vi "GDSLvClass_ReadClassColors.vi"(0 "Library Refnum":refnum<vi>, 5 "error in (no error)":errorcluster) -> (14 "Library Refnum":refnum<vi>, 15 "LvClassIconSettings":T1={"Frame"=0, "Frame thickness"=3, "Header Background"=8453954, "Header Text"=0, "ColorPublic"=16121600, "ColorProtected"=16777215, "ColorPrivate"=16777215, "Body Text"=0, "ClassBodyIcon"=""} {"Frame thickness" min=1 max=3 step=1}, 16 "LvClassIconSettingsFound":bool, 17 "ClassItemIconName(NoExtension)":string, 18 "Type":enum16{"LvClass", "Library", "X-Control"}(ring), 19 "error out":errorcluster)   [LabVIEW 2016]
uses:
  <resource>/Framework/Providers/Open_GDS/ClassProviders/Common/LvClass_class/GDSLvClass_IconSettingsType.ctl
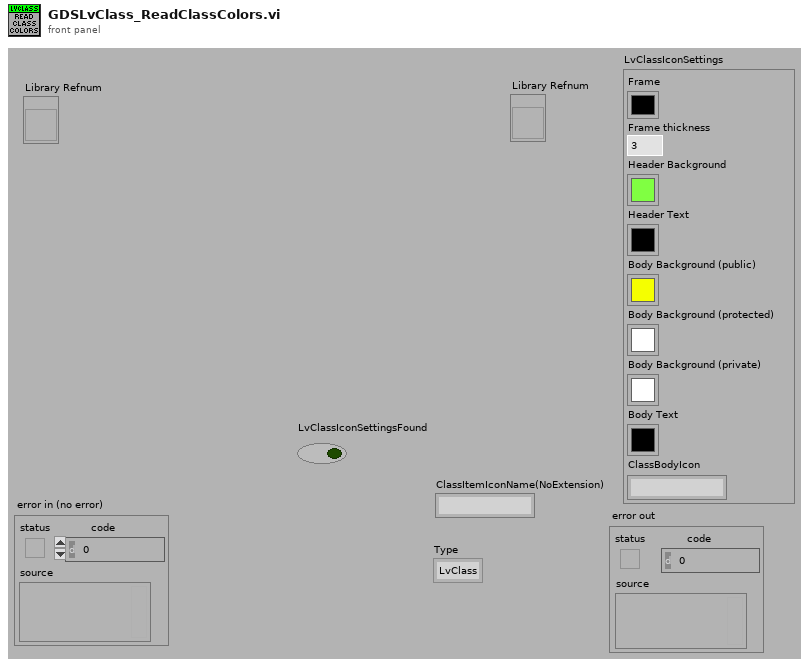
[diagram p1: front panel]
types:
  T1 = typedef "GDSLvClass_IconSettingsType.ctl" = cluster{"Frame":u32, "Frame thickness":u8, "Header Background":u32, "Header Text":u32, "ColorPublic":u32, "ColorProtected":u32, "ColorPrivate":u32, "Body Text":u32, "ClassBodyIcon":string}
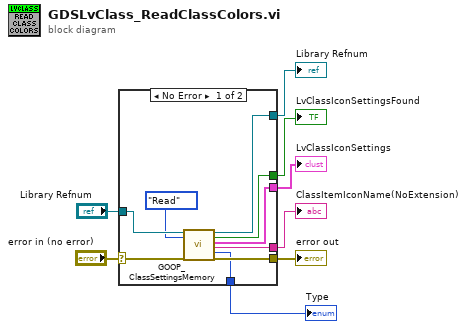
[diagram p0: block diagram]
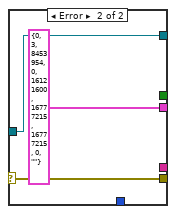
[diagram p2: hidden frame]
diagram:
  n1 = case shown="No Error" "error in (no error)" {
    selector: "error in (no error)" -> [w16 w18]
    tunnel: "Library Refnum" -> [w15 w20]
    tunnel: [w17 w20] -> w7
    tunnel: [w14 _] -> w6
    tunnel: [w12 _] -> w5
    tunnel: [w13 T1 {"Frame"=0, "Frame thickness"=3, "Header Background"=8453954, "Header Text"=0, "ColorPublic"=16121600, "ColorProtected"=16777215, "ColorPrivate"=16777215, "Body Text"=0, "ClassBodyIcon"=""} ("LvClassIconSettings")] -> w4
    tunnel: [w11 w18] -> w2
    tunnel: [w9 _] -> w1
    frame No Error {
      n2 = call <resource>:"GOOP_ClassSettingsMemory.vi"("Library Refnum"=w15, "Action"=enum16{"Read", "Write"}."Read", "error in"=w16) -> ("Library Refnum"=w17:refnum<vi>, "Found"=w14:bool, "LvClassIconSettings"=w13:T1, "ItemIcon"=w12:string, "Type"=w9:enum16{"LvClass", "Library", "X-Control"}, "error out"=w11:errorcluster)  [unwired: 11 in]
    }
    frame Error {
    }
  }
  "Library Refnum" <- w7
  "error out" <- w2
  "LvClassIconSettingsFound" <- w6
  "LvClassIconSettings" <- w4
  "ClassItemIconName(NoExtension)" <- w5
  "Type" <- w1
